vi "Select-Time (SubVI).vi"(0 "connection reference":T1, 1 "TABLE":string, 7 "COLOUM Date_Time":string, 9 "Nilainya":string, 11 "error in (no error)":errorcluster, 12 "Cari":bool) -> (4 "connection reference 2":T1, 6 "recordset data":variant[][](array[variant]), 8 "Hasil Query":string, 10 "Data":i32(listbox), 15 "error out":errorcluster)   [LabVIEW 2025]
uses:
  <vilib>/addons/database/Connection.llb/Conn ObjectReference.ctl
  <vilib>/addons/database/Connection.llb/Conn Execute.vi
  <vilib>/addons/database/Recordset.llb/Rec Fetch Recordset Data (R).vi
  <vilib>/addons/database/NI_Database_API.lvlib
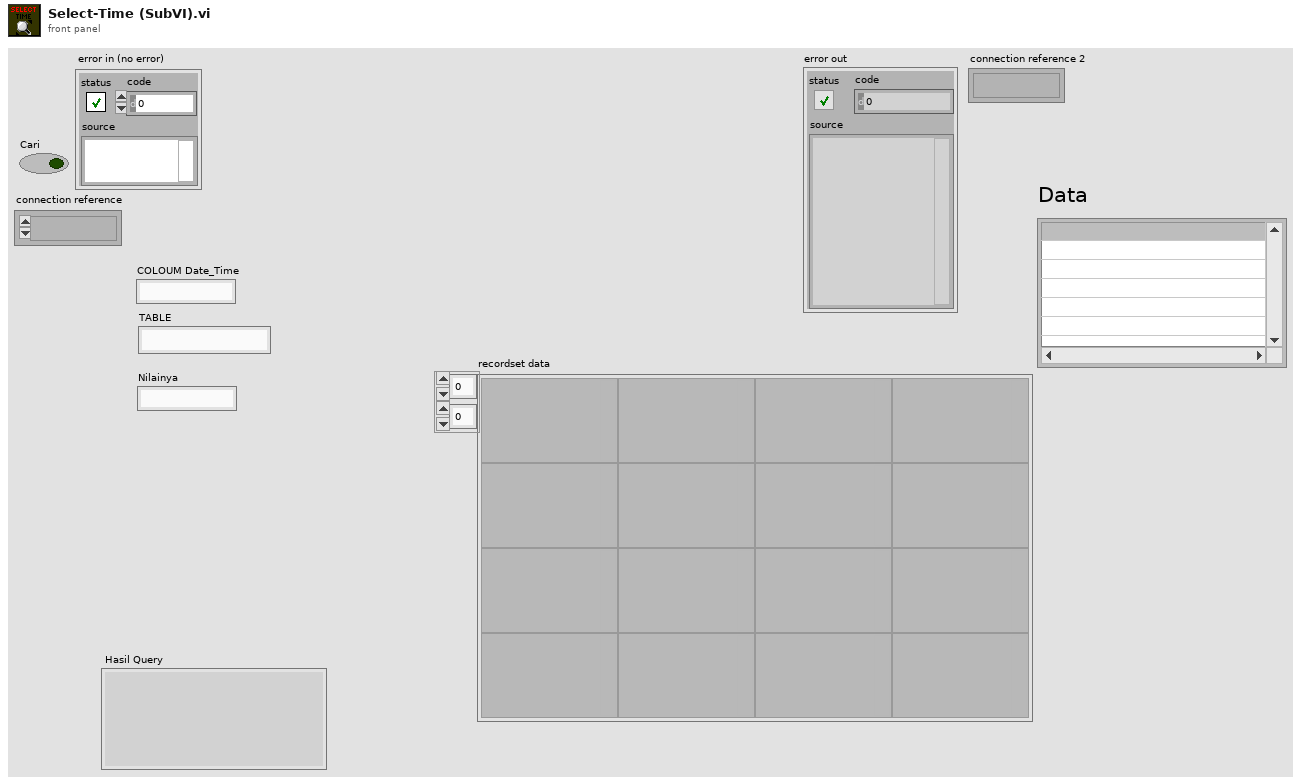
[diagram p1: front panel]
types:
  T1 = typedef "NI_Database_API.lvlib/Conn ObjectReference.ctl" = refnum<k1>
  T2 = typedef "NI_Database_API.lvlib/Rec ObjectReference.ctl" = refnum<k1>
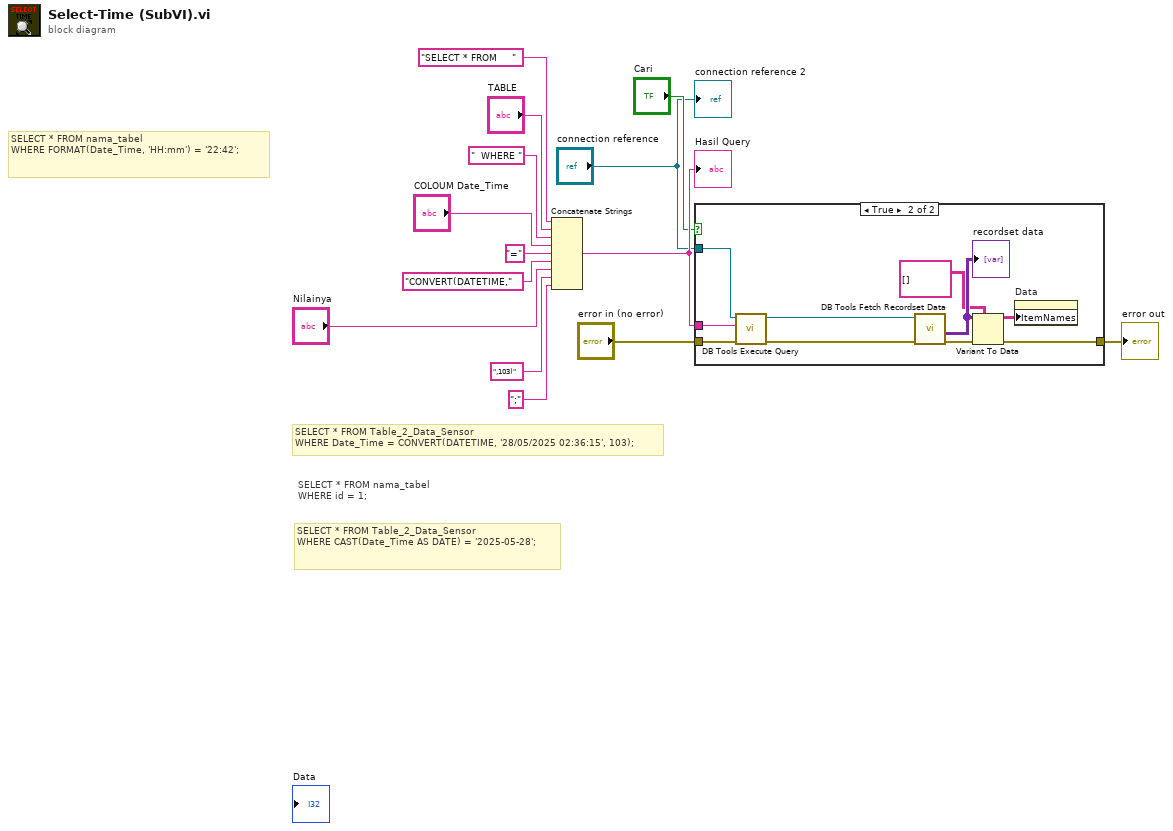
[diagram p0: block diagram]
diagram:
  # "SELECT * FROM nama_tabel\nWHERE FORMAT(Date_Time, 'HH:mm') = '22:42';"
  # "SELECT * FROM Table_2_Data_Sensor\nWHERE Date_Time = CONVERT(DATETIME, '28/05/2025 02:36:15', 103);"
  # "SELECT * FROM Table_2_Data_Sensor\nWHERE CAST(Date_Time AS DATE) = '2025-05-28';"
  # "SELECT * FROM nama_tabel\nWHERE id = 1;"
  n1 = Concatenate Strings "Concatenate Strings"("SELECT * FROM     " ("string"), "TABLE", "  WHERE " ("string"), "COLOUM Date_Time", "=" ("string"), "CONVERT(DATETIME," ("string"), "Nilainya", ",103)" ("string"), ";" ("string")) -> (w10:string)
  "Hasil Query" <- w10
  n2 = case shown="True" "Cari" {
    tunnel: w10 -> [_ w25]
    tunnel: "error in (no error)" -> [w15 w22]
    tunnel: "connection reference" -> [_ w21]
    tunnel: [w15 w16] -> w5
    frame False {
    }
    frame True {
      n3 = call-poly <vilib>:"DB Tools Execute Query.vi"("error in (no error)"=w22, "SQL query"=w25, "connection reference"=w21) -> ("error out"=w24:errorcluster, "recordset reference"=w23:T2)  [unwired: 5 in]
      n4 = call-poly <vilib>:"DB Tools Fetch Recordset Data.vi"("error in (no error)"=w24, "recordset reference"=w23) -> ("error out"=w17:errorcluster, "recordset data"=w20:variant[][])  [unwired: 3 in, 1 out]
      "recordset data" <- w20
      n5 = Variant To Data(error in=w17, type=string[][] [] ("Item Names"), Variant=w20) -> (data=w18:string[][], error out=w16:errorcluster)
      n6 = property on="Data" class="MCListbox (strict)"("ItemNames"=w18) -> ()  [unwired: 2 in, 2 out]
    }
  }
  "error out" <- w5
  "connection reference 2" <- "connection reference"
